vi "piezoGetCalibration.vi"() -> ()   [LabVIEW 2017]
uses:
  <vilib>/DAQmx/write.llb/DAQmx Write (Analog DBL 1Chan 1Samp).vi
  <vilib>/DAQmx/read.llb/DAQmx Read (Analog DBL 1Chan 1Samp).vi
  globalUtilities.vi
  <vilib>/DAQmx/create/channels.llb/DAQmx Create Channel (AO-Voltage-Basic).vi
  <vilib>/DAQmx/create/channels.llb/DAQmx Create Channel (AI-Voltage-Basic).vi
  <vilib>/DAQmx/miscellaneous.llb/DAQmx Fill In Error Info.vi
  <vilib>/Utility/file.llb/Write Delimited Spreadsheet (DBL).vi
  Piezo/lvlib/Madlib.lvlib
panel:
  out "standard output":string
  in  "piezo":i32=1 min=1 max=2
  out "set vs desired":cluster{"X":dbl, "Y":dbl}[](graph)
  in  "N":i32
  out "read vs set (BNC)":cluster{"X":dbl, "Y":dbl}[](graph)
  out "expected-read vs set BNC":cluster{"X":dbl, "Y":dbl}[](graph)
  # "SET THE POSITION VIA THE ANALOG INTERFACE AND READ IT VIA USB, TO GET THE CALIBRATION OF THE PIEZOS"
  # "These are the coefficients that have to be inserted in subvi-devices/subvi-devicesUtilites/piezoPositionToVoltage.vi\nThe lonely \"2\" is the power of x (the terms are a*x^2 + b*x + c)\nThe top one is for um -> V, the bottom one V->um."
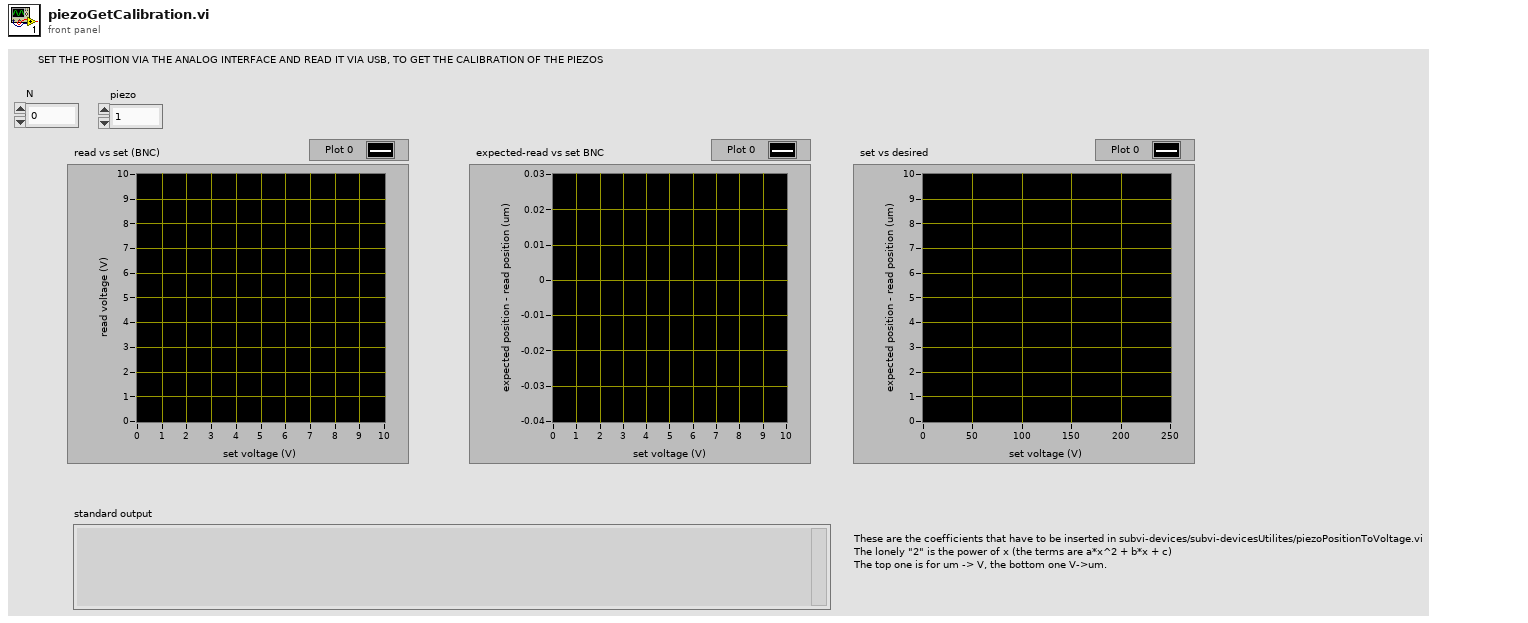
[diagram p1: front panel]
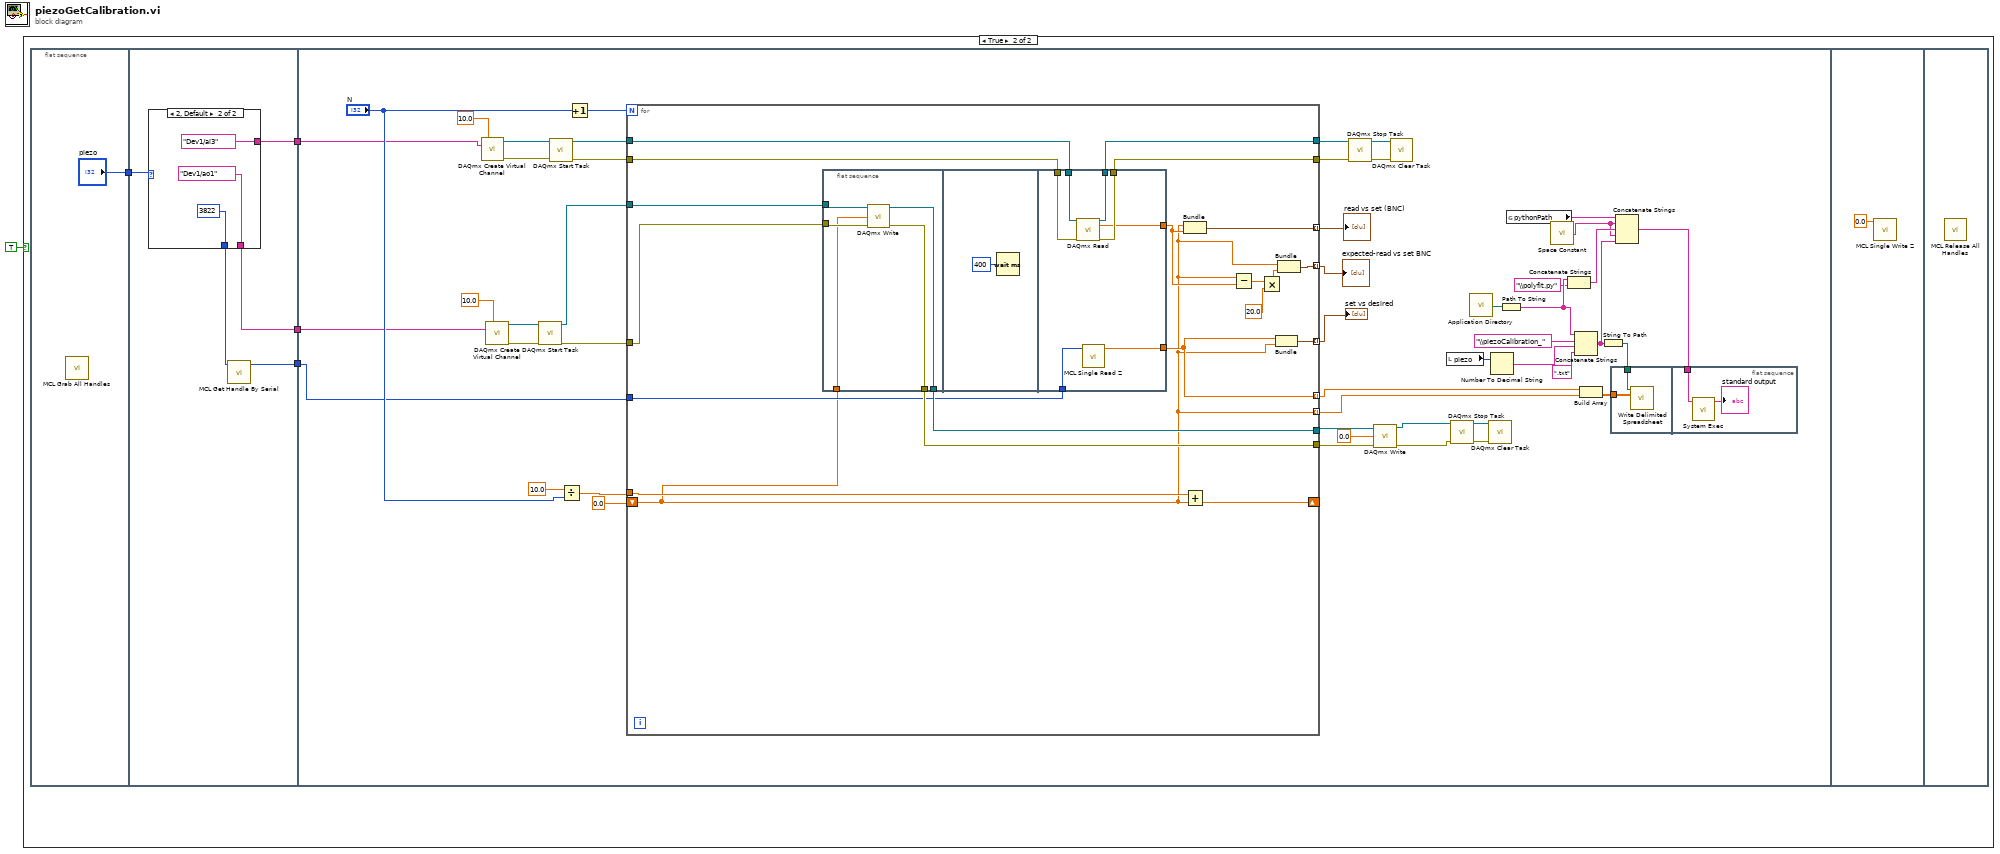
[diagram p0: block diagram]
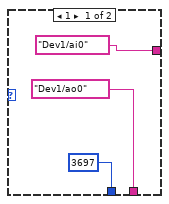
[diagram p3: hidden frame]
diagram:
  n1 = case shown="True" TRUE {
    frame False {
    }
    frame True {
      n2 = flat-sequence {
        tunnel: ["piezo"] -> w4
        tunnel: [w11] -> w5
        tunnel: w4 -> [w10]
        tunnel: [w9] -> w3
        tunnel: [w8] -> w2
        tunnel: w5 -> [w37]
        tunnel: w3 -> [w32]
        tunnel: w2 -> [w33]
        frame #0 {
          n3 = call "MCL Grab All Handles.vi"() -> ()  [unwired: 11 in, 1 out]
        }
        frame #1 {
          n4 = case shown="2, Default" w10 {
            tunnel: [tag "Dev1/ai0" ("physical channels") tag "Dev1/ai3" ("physical channels")] -> w9
            tunnel: [tag "Dev1/ao0" ("physical channels") tag "Dev1/ao1" ("physical channels")] -> w8
            tunnel: [i16 3697 ("serial") i16 3822 ("serial")] -> w7
            frame 1 {
            }
            frame 2, Default {
            }
          }
          n5 = call "MCL Get Handle By Serial.vi"("serial"=w7) -> ("function return"=w11:i32)  [unwired: 10 in]
        }
        frame #2 {
          n6 = call-poly <vilib>:"DAQmx Create Virtual Channel.vi"("maximum value"=10.0, "physical channels"=w32) -> ("task out"=w65:refnum<k21>, "error out"=w64:errorcluster)  [unwired: 12 in]
          n7 = call-poly <vilib>:"DAQmx Create Virtual Channel.vi"("maximum value"=10.0, "physical channels"=w33) -> ("task out"=w48:refnum<k21>, "error out"=w47:errorcluster)  [unwired: 12 in]
          n8 = call <vilib>:"DAQmx Start Task.vi"("task/channels in"=w48, "error in"=w47) -> ("task out"=w46:refnum<k21>, "error out"=w45:errorcluster)  [unwired: 12 in]
          n9 = call <vilib>:"DAQmx Start Task.vi"("task/channels in"=w65, "error in"=w64) -> ("task out"=w63:refnum<k21>, "error out"=w62:errorcluster)  [unwired: 12 in]
          n10 = Divide(x=10.0, y="N") -> (x/y=w55:dbl)
          n11 = Increment(x="N") -> (x+1=w52:i32)
          n12 = for {
            N: w52 -> [_]
            tunnel: w63 -> [w89]
            tunnel: w62 -> [w88]
            tunnel: [w87] -> w61
            tunnel: [w86] -> w60
            tunnel: w55 -> [w85]
            shift-right: [w83] -> _
            shift-left: 0.0 -> [w70]
            tunnel: [w84] -> w51 mode=indexing
            tunnel: [w82] -> w50 mode=indexing
            tunnel: w46 -> [w77]
            tunnel: w45 -> [w76]
            tunnel: [w75] -> w42
            tunnel: [w74] -> w41
            tunnel: w37 -> [w73]
            tunnel: [w72] -> w36 mode=indexing
            tunnel: [w71] -> w35 mode=indexing
            tunnel: [w70] -> w34 mode=indexing
            n13 = flat-sequence {
              tunnel: w70 -> [w90]
              tunnel: w77 -> [w94]
              tunnel: w76 -> [w93]
              tunnel: [w92] -> w75
              tunnel: [w91] -> w74
              tunnel: w89 -> [w102]
              tunnel: w88 -> [w101]
              tunnel: [w100] -> w87
              tunnel: [w99] -> w86
              tunnel: [w98] -> w80
              tunnel: w73 -> [w97]
              tunnel: [w96] -> w71
              frame #0 {
                n14 = call-poly <vilib>:"DAQmx Write.vi"("task/channels in"=w94, "data"=w90, "error in"=w93) -> ("task out"=w92:refnum<k21>, "error out"=w91:errorcluster)  [unwired: 10 in, 1 out]
              }
              frame #1 {
                n15 = Wait (ms)(milliseconds to wait=u32 400) -> ()  [unwired: 1 out]
              }
              frame #2 {
                n16 = call-poly <vilib>:"DAQmx Read.vi"("task/channels in"=w102, "error in"=w101) -> ("task out"=w100:refnum<k21>, "data"=w98:dbl, "error out"=w99:errorcluster)  [unwired: 11 in]
                n17 = call "MCL Single Read Z.vi"("handle"=w97) -> ("function return"=w96:dbl)  [unwired: 10 in]
              }
            }
            n18 = Bundle(w70, "data"=w80) -> (w84:cluster{dbl, "data":dbl})  [unwired: 1 in]
            n19 = Add(x=w85, y=w70) -> (x+y=w83:dbl)
            n20 = Subtract(x=w70, y=w80) -> (x-y=w81:dbl)
            n21 = Multiply(x=w81, y=20.0) -> (x*y=w79:dbl)
            n22 = Bundle("function return"=w71, w70) -> (w72:cluster{"function return":dbl, dbl})  [unwired: 1 in]
            n23 = Bundle(w70, w79) -> (w82:cluster{dbl, dbl})  [unwired: 1 in]
          }
          "read vs set (BNC)" <- w51
          "expected-read vs set BNC" <- w50
          "set vs desired" <- w36
          n24 = call <vilib>:"DAQmx Stop Task.vi"("task/channels in"=w61, "error in"=w60) -> ("task out"=w59:refnum<k21>, "error out"=w58:errorcluster)  [unwired: 12 in]
          n25 = call-poly <vilib>:"DAQmx Write.vi"("task/channels in"=w42, "data"=0.0, "error in"=w41) -> ("task out"=w40:refnum<k21>, "error out"=w39:errorcluster)  [unwired: 10 in, 1 out]
          n26 = call <vilib>:"DAQmx Clear Task.vi"("task in"=w59, "error in"=w58) -> ()  [unwired: 13 in, 1 out]
          n27 = local read "piezo"() -> (w29:i32)
          n28 = call <vilib>:"DAQmx Stop Task.vi"("task/channels in"=w40, "error in"=w39) -> ("task out"=w43:refnum<k21>, "error out"=w44:errorcluster)  [unwired: 12 in]
          n29 = call <vilib>:"Application Directory.vi"() -> ("Application Directory"=w19:path)
          n30 = call <vilib>:"DAQmx Clear Task.vi"("task in"=w43, "error in"=w44) -> ()  [unwired: 13 in, 1 out]
          n31 = Number To Decimal String(number=w29) -> (decimal integer string=w28:string)  [unwired: 1 in]
          n32 = Path To String(path=w19) -> (string=w24:string)
          n33 = global read "globalUtilities.vi" "pythonPath"() -> (w25:string)
          n34 = call <vilib>:"Space Constant.vi"() -> ("String"=w21:string)
          n35 = Concatenate Strings(w24, "\\polyfit.py" ("string")) -> (w22:string)
          n36 = Concatenate Strings(w24, "\\piezoCalibration_", w28, ".txt" ("string")) -> (w20:string)
          n37 = Build Array(w35, w34) -> (w31:dbl[][])
          n38 = String To Path(string=w20) -> (path=w27:path)
          n39 = flat-sequence {
            tunnel: w31 -> [w67]
            tunnel: w27 -> [w66]
            tunnel: w18 -> [w68]
            frame #0 {
              n40 = call-poly <vilib>:"Write Delimited Spreadsheet.vi"("file path (dialog if empty)"=w66, "2D data"=w67) -> ()  [unwired: 12 in, 2 out]
            }
            frame #1 {
              n41 = call <vilib>:"System Exec.vi"("command line"=w68) -> ("standard output"=→"standard output":string)  [unwired: 7 in, 3 out]
            }
          }
          n42 = Concatenate Strings(w25, w21, w22, w21, w20) -> (w18:string)
        }
        frame #3 {
          n43 = call "MCL Single Write Z.vi"("position"=0.0) -> ()  [unwired: 10 in, 1 out]
        }
        frame #4 {
          n44 = call "MCL Release All Handles.vi"() -> ()  [unwired: 12 in]
        }
      }
    }
  }
